vi "Set CPU.vi"(8 "error in (no error)":errorcluster, 10 "CPU Info":refnum<class "CPU Info.lvclass">, 11 "Hardware Info in":refnum<class "Hardware Info.lvclass">) -> (0 "error out":errorcluster, 3 "Hardware Info out":refnum<class "Hardware Info.lvclass">)   [LabVIEW 2017, in "DSF Core.lvlib" / "Hardware Info.lvclass"]
uses:
  Hardware Info/Hardware Info.lvclass
  CPU Info/CPU Info.lvclass
  Hardware Info/Hardware Info.lvclass/Hardware Info.ctl
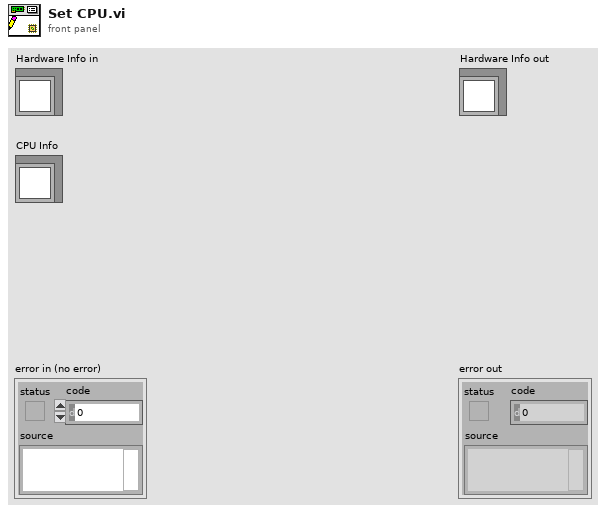
[diagram p1: front panel]
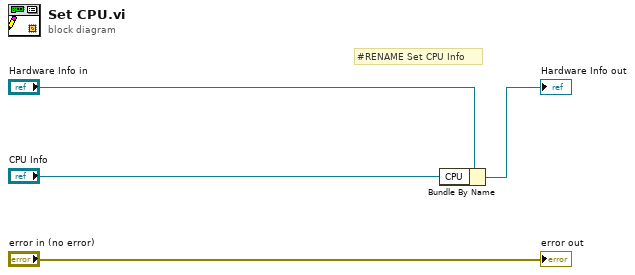
[diagram p0: block diagram]
diagram:
  # "#RENAME Set CPU Info"
  n1 = Bundle By Name(cluster="Hardware Info in", "CPU"="CPU Info") -> (→"Hardware Info out":refnum<class "Hardware Info.lvclass">)
  "error out" <- "error in (no error)"
